vi "main screen V2.vi"() -> ()   [LabVIEW 2020]
uses:
  <vilib>/userdefined/High Color/IMAQdx.ctl
  <vilib>/DAQmx/read.llb/DAQmx Read (Analog 1D DBL NChan 1Samp).vi
  <vilib>/DAQmx/create/channels.llb/DAQmx Create Channel (AI-Voltage-Basic).vi
  <vilib>/DAQmx/create/channels.llb/DAQmx Create Channel (AI-Temperature-Thermocouple).vi
  <vilib>/DAQmx/configure/timing.llb/DAQmx Timing (Sample Clock).vi
  <vilib>/DAQmx/miscellaneous.llb/DAQmx Fill In Error Info.vi
  <vilib>/Utility/file.llb/Write Delimited Spreadsheet (string).vi
  <vilib>/Utility/file.llb/Write Delimited Spreadsheet (DBL).vi
  <vilib>/vision/driver/NI_Vision_Acquisition_Software.lvlib
  <resource>/objmgr/imaqdx.rc
  <resource>/objmgr/daqmx.rc
panel:
  out "Saving Data":bool
  out "System Time":dbl
  in  "Sample Rate":dbl=90.0
  out "error out 2":errorcluster
  out "Image 2":T1(plugin-control)
  out "Image":T1(plugin-control)
  out "error out":errorcluster
  out "Clock":dbl[](graph)
  out "T.C 2":dbl[](graph)
  out "T.C 3":dbl[](graph)
  out "T.C 4":dbl[](graph)
  out "T.C 5":dbl[](graph)
  out "T.C 6":dbl[](graph)
  out "T.C 7":dbl[](graph)
  out "Front Diode":dbl[](graph)
  out "Rear Diode":dbl[](graph)
  out "T.C 1":dbl[](graph)
  out "T.C 8":dbl[](graph)
  in  "stop":bool
  in  "physical channels":tag="cDAQ1Mod1/ai1,cDAQ1Mod1/ai2"
  in  "TC channel":tag="cDAQ1Mod3/ai0,cDAQ1Mod3/ai1,cDAQ1Mod3/ai2,cDAQ1Mod3/ai3,cDAQ1Mod3/ai4,cDAQ1Mod3/ai5,cDAQ1Mod3/ai6,cDAQ1Mod3/ai7"
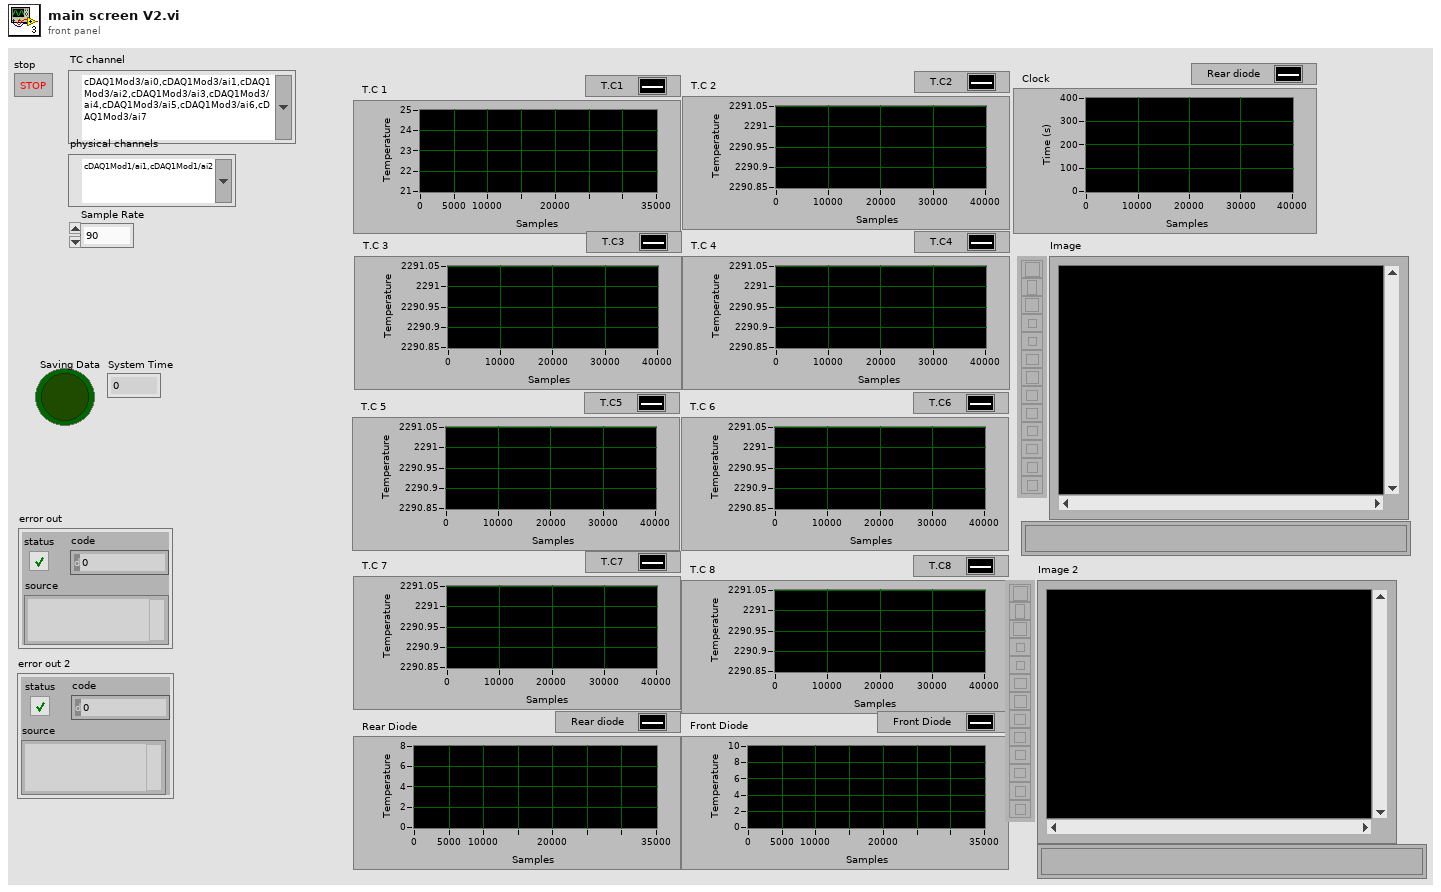
[diagram p1: front panel]
types:
  T1 = typedef "IMAQ Image.ctl" = refnum<image>
  T2 = typedef "IMAQdx.ctl" = refnum<k21>
  T3 = typedef "IMAQ AVI2 Refnum.ctl" = refnum<k20>
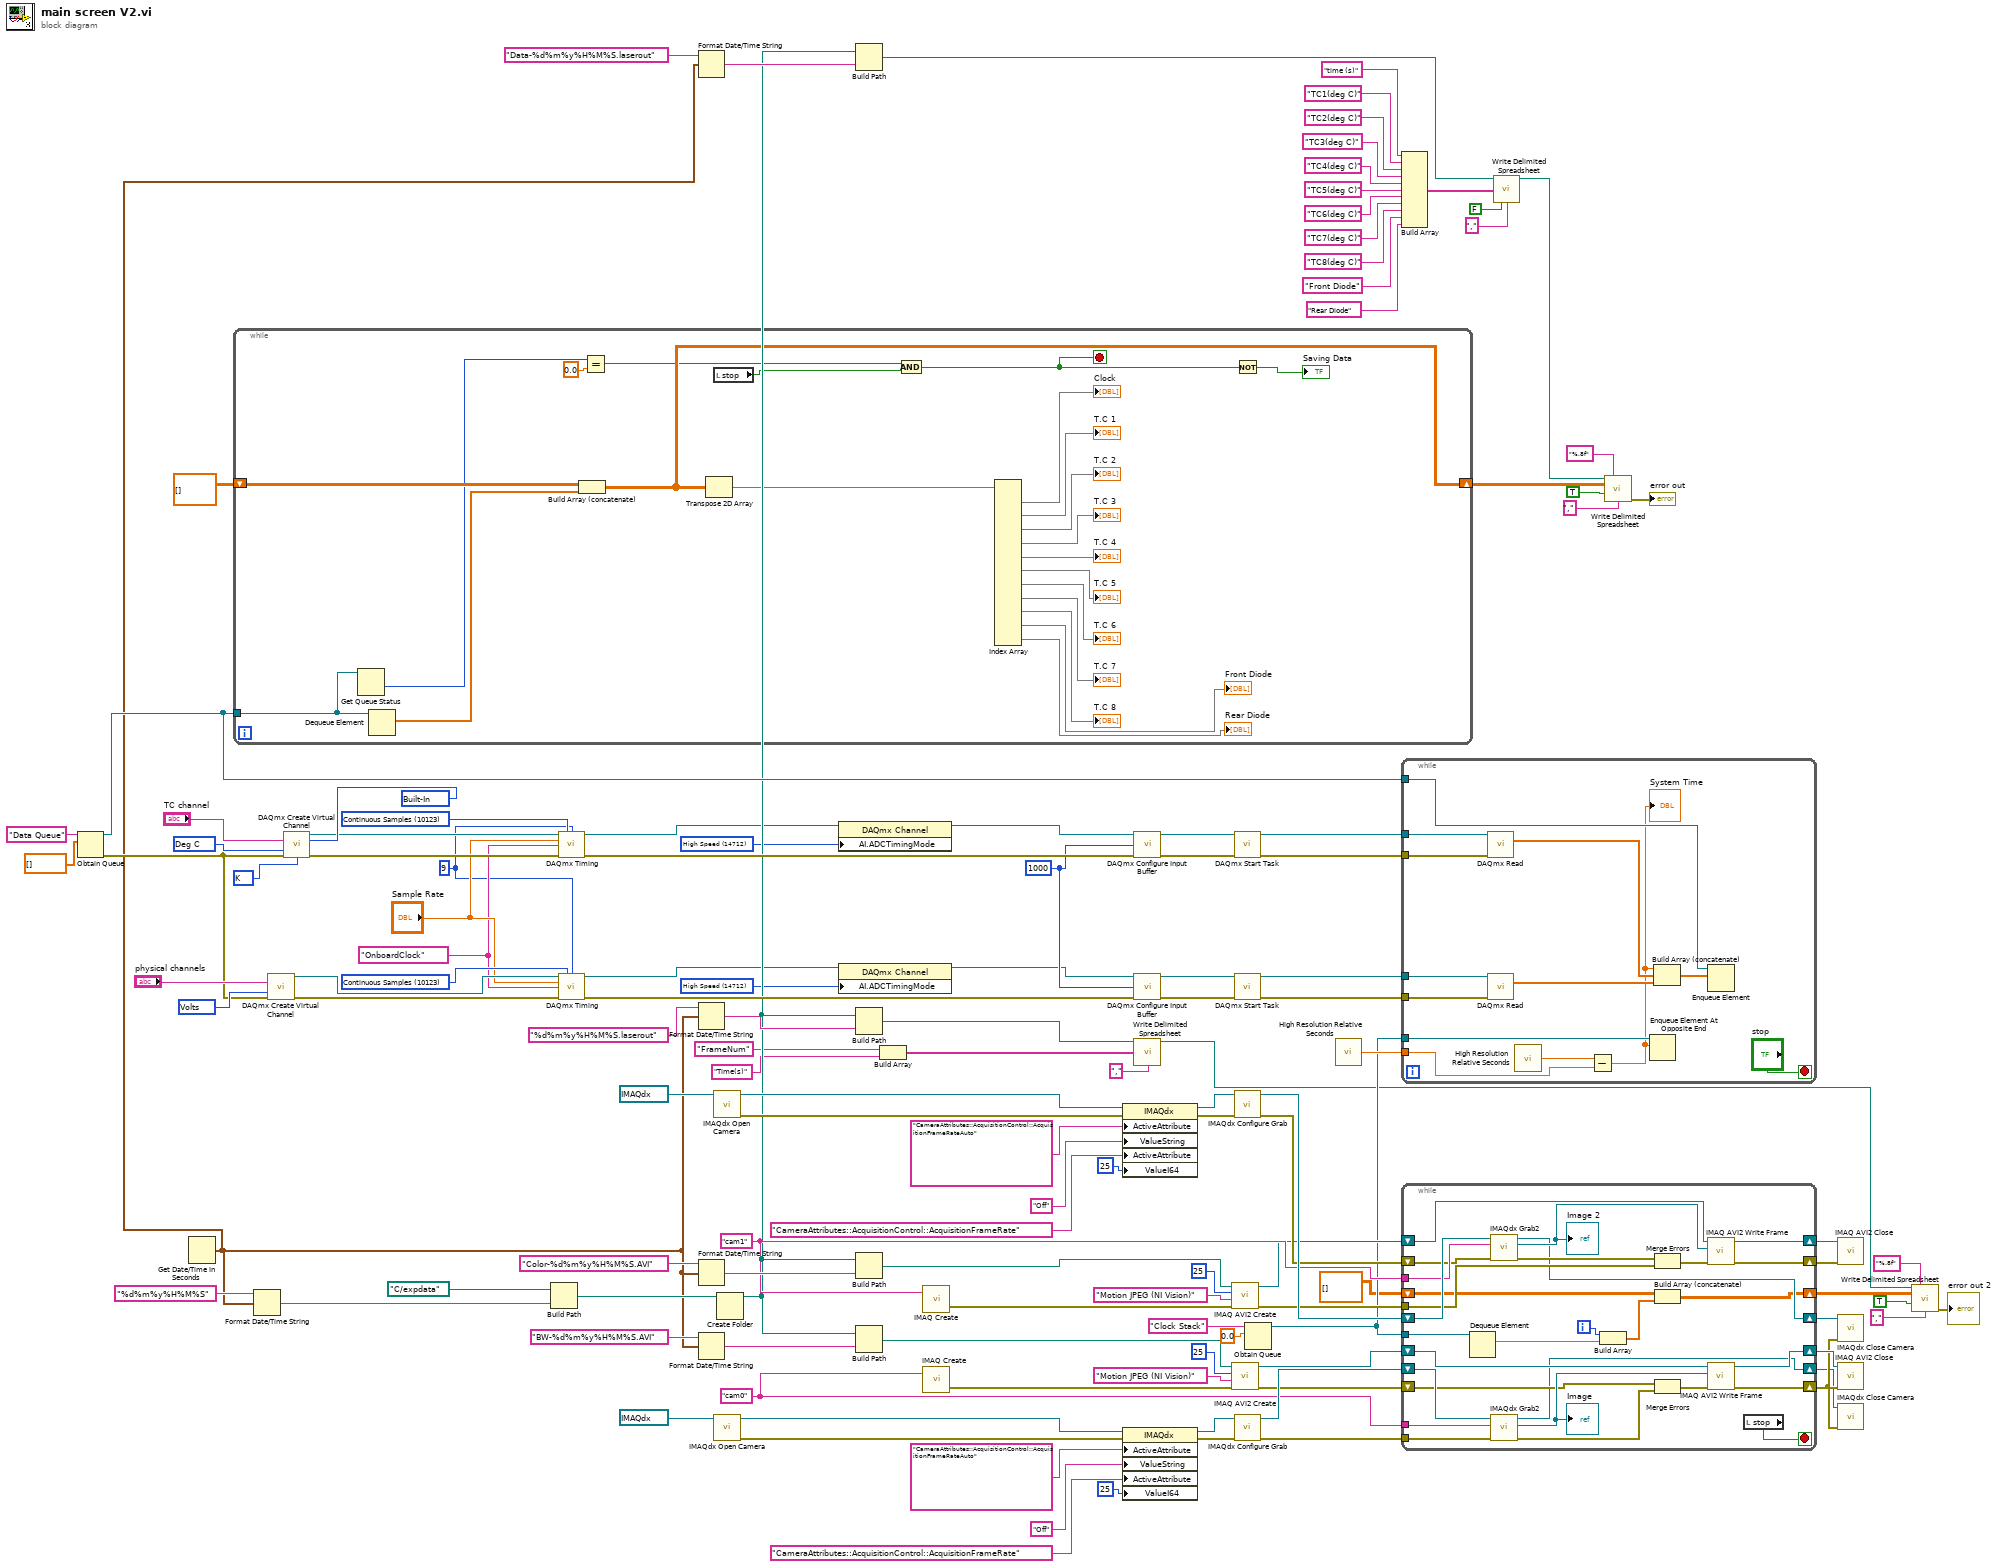
[diagram p0: block diagram]
diagram:
  w1 = 14712 items=["Automatic"=16097, "High Resolution"=10195, "High Speed"=14712, "Best 50 Hz Rejection"=14713, "Best 60 Hz Rejection"=14714, "Custom"=10137] ("AI.ADCTimingMode")
  w4 = 14712 items=["Automatic"=16097, "High Resolution"=10195, "High Speed"=14712, "Best 50 Hz Rejection"=14713, "Best 60 Hz Rejection"=14714, "Custom"=10137] ("AI.ADCTimingMode")
  w7 = 9 ("samples per channel")
  w8 = tag "OnboardClock" ("source")
  w44 = "cam1" ("Image Name")
  w38 = "cam0" ("Image Name")
  w105 = u32 1000 ("buffer size (in samples per channel)")
  w117 = 10123 items=["Finite Samples"=10178, "Continuous Samples"=10123, "Hardware Timed Single Point"=12522] ("sample mode")
  w118 = 10123 items=["Finite Samples"=10178, "Continuous Samples"=10123, "Hardware Timed Single Point"=12522] ("sample mode")
  w119 = 10073 items=["J"=10072, "K"=10073, "N"=10077, "R"=10082, "S"=10085, "T"=10086, "B"=10047, "E"=10055] ("thermocouple type")
  w123 = 10348 items=["Volts"=10348, "From Custom Scale"=10065] ("units")
  w125 = 10200 items=["Built-In"=10200, "Constant Value"=10116, "Channel"=10113] ("cjc source")
  w126 = 10143 items=["Deg C"=10143, "Deg F"=10144, "Kelvins"=10325, "Deg R"=10145, "From Custom Scale"=10065] ("units")
  n1 = Obtain Queue(name (unnamed)="Data Queue", element data type=dbl[] []) -> (queue out=w130:refnum<queue>, error out=w77:errorcluster)  [unwired: 3 in, 1 out]
  n2 = Get Date/Time In Seconds() -> (seconds since 1Jan1904=w25:timestamp)
  n3 = while {
    tunnel: w130 -> [w135]
    shift-right: [w139] -> w80
    shift-left: dbl[][] [] -> [w152]
    stop <- w132 stop-if-true
    n4 = Get Queue Status(queue=w135) -> (# pending insert=w134:i32)  [unwired: 2 in, 7 out]
    n5 = Dequeue Element(queue=w135) -> (element=w151:dbl[])  [unwired: 2 in, 3 out]
    n6 = Build Array (concatenate)(w152, w151) -> (w139:dbl[][])
    n7 = Equal?(x=w134, y=0.0) -> (x = y?=w137:bool)
    n8 = Transpose 2D Array(2D array=w139) -> (transposed array=w138:dbl[][])
    n9 = local read "stop"() -> (w133:bool)
    n10 = And(x=w137, y=w133) -> (x .and. y?=w132:bool)
    n11 = Index Array(array=w138) -> (element #1=→"Clock":dbl[], element #2=→"T.C 1":dbl[], element #3=→"T.C 2":dbl[], element #4=→"T.C 3":dbl[], element #5=→"T.C 4":dbl[], element #6=→"T.C 5":dbl[], element #7=→"T.C 6":dbl[], element #8=→"T.C 7":dbl[], element #9=→"T.C 8":dbl[], element #10=→"Front Diode":dbl[], element #11=→"Rear Diode":dbl[])  [unwired: 22 in]
    n12 = Not(x=w132) -> (.not. x?=→"Saving Data":bool)
  }
  n13 = Format Date/Time String(time format string (%c)="%d%m%y%H%M%S", seconds (now)=w25) -> (date/time string=w101:string)  [unwired: 1 in]
  n14 = call-poly <vilib>:"DAQmx Create Virtual Channel.vi"("physical channels"="physical channels", "units"=w123, "error in"=w77) -> ("task out"=w122:refnum<k21>, "error out"=w76:errorcluster)  [unwired: 11 in]
  n15 = call-poly <vilib>:"DAQmx Create Virtual Channel.vi"("physical channels"="TC channel", "cjc source"=w125, "units"=w126, "error in"=w77, "thermocouple type"=w119) -> ("task out"=w121:refnum<k21>, "error out"=w120:errorcluster)  [unwired: 9 in]
  n16 = Build Path(base path=path "C:/expdata", name or relative path=w101) -> (appended path=w100:path)
  n17 = call-poly <vilib>:"DAQmx Timing.vi"("task/channels in"=w121, "sample mode"=w118, "samples per channel"=w7, "rate"="Sample Rate", "source"=w8, "error in"=w120) -> ("task out"=w3:refnum<k21>, "error out"=w115:errorcluster)  [unwired: 8 in]
  n18 = call-poly <vilib>:"DAQmx Timing.vi"("task/channels in"=w122, "sample mode"=w117, "samples per channel"=w7, "rate"="Sample Rate", "source"=w8, "error in"=w76) -> ("task out"=w6:refnum<k21>, "error out"=w116:errorcluster)  [unwired: 8 in]
  n19 = Format Date/Time String(time format string (%c)="Data-%d%m%y%H%M%S.laserout", seconds (now)=w25) -> (date/time string=w98:string)  [unwired: 1 in]
  n20 = Format Date/Time String(time format string (%c)="%d%m%y%H%M%S.laserout", seconds (now)=w25) -> (date/time string=w24:string)  [unwired: 1 in]
  n21 = Format Date/Time String(time format string (%c)="Color-%d%m%y%H%M%S.AVI", seconds (now)=w25) -> (date/time string=w49:string)  [unwired: 1 in]
  n22 = Format Date/Time String(time format string (%c)="BW-%d%m%y%H%M%S.AVI", seconds (now)=w25) -> (date/time string=w52:string)  [unwired: 1 in]
  n23 = call <vilib>:"IMAQdx Open Camera.vi"("Session In"=T2 "cam1") -> ("error out"=w63:errorcluster, "Session Out"=w65:T2)  [unwired: 9 in]
  n24 = call <vilib>:"IMAQdx Open Camera.vi"("Session In"=T2 "cam0") -> ("error out"=w72:errorcluster, "Session Out"=w74:T2)  [unwired: 9 in]
  n25 = Create Folder(path (use dialog)=w100) -> (created path=w23:path)  [unwired: 2 in, 2 out]
  n26 = property class="DAQmx Channel"(reference=w3, "AI.ADCTimingMode"=w1) -> (reference out=w2:refnum<k21>)  [unwired: 1 in, 1 out]
  n27 = property class="DAQmx Channel"(reference=w6, "AI.ADCTimingMode"=w4) -> (reference out=w5:refnum<k21>)  [unwired: 1 in, 1 out]
  n28 = Build Path(base path=w23, name or relative path=w98) -> (appended path=w86:path)
  n29 = Build Path(base path=w23, name or relative path=w24) -> (appended path=w22:path)
  n30 = Build Path(base path=w23, name or relative path=w49) -> (appended path=w48:path)
  n31 = Build Path(base path=w23, name or relative path=w52) -> (appended path=w51:path)
  n32 = Build Array("FrameNum", "Time(s)") -> (w18:string[])
  n33 = call "IMAQ Create"("Image Name"=w44) -> ("error out"=w56:errorcluster)  [unwired: 4 in, 1 out]
  n34 = call "IMAQ Create"("Image Name"=w38) -> ("error out"=w55:errorcluster)  [unwired: 4 in, 1 out]
  n35 = property class="IMAQdx"(reference=w65, error in=w63, "ActiveAttribute"="CameraAttributes::AcquisitionControl::AcquisitionFrameRateAuto", "ValueString"="Off", "ActiveAttribute"="CameraAttributes::AcquisitionControl::AcquisitionFrameRate", "ValueI64"=u32 25 ("ValueU32")) -> (reference out=w64:T2, error out=w62:errorcluster)
  n36 = property class="IMAQdx"(reference=w74, error in=w72, "ActiveAttribute"="CameraAttributes::AcquisitionControl::AcquisitionFrameRateAuto", "ValueString"="Off", "ActiveAttribute"="CameraAttributes::AcquisitionControl::AcquisitionFrameRate", "ValueI64"=u32 25 ("ValueU32")) -> (reference out=w73:T2, error out=w71:errorcluster)
  n37 = call <vilib>:"DAQmx Configure Input Buffer.vi"("task/channels in"=w2, "buffer size (in samples per channel)"=w105, "error in"=w115) -> ("task out"=w113:refnum<k21>, "error out"=w111:errorcluster)  [unwired: 11 in]
  n38 = call <vilib>:"DAQmx Configure Input Buffer.vi"("task/channels in"=w5, "buffer size (in samples per channel)"=w105, "error in"=w116) -> ("task out"=w109:refnum<k21>, "error out"=w106:errorcluster)  [unwired: 11 in]
  n39 = call-poly <vilib>:"Write Delimited Spreadsheet.vi"("file path (dialog if empty)"=w22, "1D data"=w18, "delimiter (\\t)"="," ("delimiter (\\t)")) -> ("new file path (Not A Path if cancelled)"=w14:path)  [unwired: 11 in, 1 out]
  n40 = call "IMAQ AVI2 Create"("error in (no error)"=w56, "Codec"="Motion JPEG (NI Vision)", "Frames Per Second"=u32 25, "AVI Path"=w48) -> ("error out"=w41:errorcluster, "AVI Refnum"=w42:T3)  [unwired: 6 in]
  n41 = call "IMAQ AVI2 Create"("error in (no error)"=w55, "Codec"="Motion JPEG (NI Vision)", "Frames Per Second"=u32 25, "AVI Path"=w51) -> ("error out"=w36:errorcluster, "AVI Refnum"=w37:T3)  [unwired: 6 in]
  n42 = call <vilib>:"DAQmx Start Task.vi"("task/channels in"=w113, "error in"=w111) -> ("task out"=w112:refnum<k21>, "error out"=w110:errorcluster)  [unwired: 12 in]
  n43 = call <vilib>:"DAQmx Start Task.vi"("task/channels in"=w109, "error in"=w106) -> ("task out"=w108:refnum<k21>, "error out"=w107:errorcluster)  [unwired: 12 in]
  n44 = call <vilib>:"IMAQdx Configure Grab.vi"("error in"=w62, "Session In"=w64) -> ("error out"=w43:errorcluster, "Session Out"=w45:T2)  [unwired: 8 in]
  n45 = call <vilib>:"IMAQdx Configure Grab.vi"("error in"=w71, "Session In"=w73) -> ("error out"=w39:errorcluster, "Session Out"=w40:T2)  [unwired: 8 in]
  n46 = Obtain Queue(name (unnamed)="Clock Stack", element data type=0.0) -> (queue out=w27:refnum<queue>)  [unwired: 3 in, 2 out]
  n47 = call <vilib>:"High Resolution Relative Seconds.vi"() -> ("relative seconds"=w114:dbl)
  n48 = Build Array("time (s)", "TC1(deg C)", "TC2(deg C)", "TC3(deg C)", "TC4(deg C)", "TC5(deg C)", "TC6(deg C)", "TC7(deg C)", "TC8(deg C)", "Front Diode", "Rear Diode") -> (w85:string[])
  n49 = while {
    tunnel: w130 -> [w165]
    tunnel: w112 -> [w164]
    tunnel: w110 -> [w163]
    tunnel: w108 -> [w162]
    tunnel: w107 -> [w161]
    tunnel: w114 -> [w160]
    tunnel: w27 -> [w154]
    stop <- "stop" stop-if-true
    n50 = call-poly <vilib>:"DAQmx Read.vi"("task/channels in"=w164, "error in"=w163) -> ("data"=w158:dbl[])  [unwired: 11 in, 2 out]
    n51 = call-poly <vilib>:"DAQmx Read.vi"("task/channels in"=w162, "error in"=w161) -> ("data"=w157:dbl[])  [unwired: 11 in, 2 out]
    n52 = call <vilib>:"High Resolution Relative Seconds.vi"() -> ("relative seconds"=w159:dbl)
    n53 = Subtract(x=w159, y=w160) -> (x-y=w153:dbl)
    "System Time" <- w153
    n54 = Enqueue Element At Opposite End(queue=w154, element=w153) -> ()  [unwired: 2 in, 3 out]
    n55 = Build Array (concatenate)(w153, w158, w157) -> (w156:dbl[])
    n56 = Enqueue Element(queue=w165, element=w156) -> ()  [unwired: 2 in, 3 out]
  }
  n57 = while {
    tunnel: w44 -> [w191]
    tunnel: w41 -> [w186]
    tunnel: w39 -> [w184]
    tunnel: w38 -> [w183]
    shift-right: [w174] -> w31
    shift-left: w45 -> [w192]
    shift-right: [w176] -> w33
    shift-left: w43 -> [w190]
    shift-right: [w178] -> w35
    shift-left: w42 -> [w189]
    shift-right: [w173] -> w30
    shift-left: w40 -> [w185]
    shift-right: [w177] -> w34
    shift-left: w37 -> [w182]
    shift-right: [w175] -> w32
    shift-left: w36 -> [w180]
    tunnel: w27 -> [w172]
    shift-right: [w169] -> w13
    shift-left: dbl[][] [] -> [w170]
    i -> [w167]
    stop <- w168 stop-if-true
    n58 = Dequeue Element(queue=w172) -> (element=w166:dbl)  [unwired: 2 in, 3 out]
    n59 = call <vilib>:"IMAQdx Grab2.vi"("error in"=w190, "Image In"=w191, "Session In"=w192) -> ("error out"=w187:errorcluster, "Image Out"=w193:T1, "Session Out"=w174:T2)  [unwired: 5 in, 1 out]
    "Image 2" <- w193
    n60 = call <vilib>:"IMAQdx Grab2.vi"("error in"=w184, "Image In"=w183, "Session In"=w185) -> ("error out"=w181:errorcluster, "Image Out"=w194:T1, "Session Out"=w173:T2)  [unwired: 5 in, 1 out]
    "Image" <- w194
    n61 = Build Array(w167, w166) -> (w171:dbl[])
    n62 = Merge Errors(w187, w186) -> (w188:errorcluster)
    n63 = Build Array (concatenate)(w170, w171) -> (w169:dbl[][])
    n64 = Merge Errors(w180, w181) -> (w179:errorcluster)
    n65 = call "IMAQ AVI2 Write Frame"("error in (no error)"=w188, "Image"=w193, "AVI Refnum"=w189) -> ("error out"=w176:errorcluster, "AVI Refnum (duplicate)"=w178:T3)  [unwired: 6 in, 1 out]
    n66 = call "IMAQ AVI2 Write Frame"("error in (no error)"=w179, "Image"=w194, "AVI Refnum"=w182) -> ("error out"=w175:errorcluster, "AVI Refnum (duplicate)"=w177:T3)  [unwired: 6 in, 1 out]
    n67 = local read "stop"() -> (w168:bool)
  }
  n68 = call-poly <vilib>:"Write Delimited Spreadsheet.vi"("file path (dialog if empty)"=w86, "1D data"=w85, "transpose? (no:F)"=FALSE, "delimiter (\\t)"="," ("delimiter (\\t)")) -> ("new file path (Not A Path if cancelled)"=w79:path)  [unwired: 10 in, 1 out]
  n69 = call-poly <vilib>:"Write Delimited Spreadsheet.vi"("file path (dialog if empty)"=w79, "format (%.3f)"="%.8f", "2D data"=w80, "append to file? (new file:F)"=TRUE, "delimiter (\\t)"="," ("delimiter (\\t)")) -> ("error out"=→"error out":errorcluster)  [unwired: 9 in, 1 out]
  n70 = call "IMAQ AVI2 Close"("error in (no error)"=w33, "AVI Refnum"=w35) -> ()  [unwired: 9 in, 1 out]
  n71 = call <vilib>:"IMAQdx Close Camera.vi"("error in"=w32, "Session In"=w31) -> ()  [unwired: 9 in, 1 out]
  n72 = call "IMAQ AVI2 Close"("error in (no error)"=w32, "AVI Refnum"=w34) -> ()  [unwired: 9 in, 1 out]
  n73 = call <vilib>:"IMAQdx Close Camera.vi"("error in"=w32, "Session In"=w30) -> ()  [unwired: 9 in, 1 out]
  n74 = call-poly <vilib>:"Write Delimited Spreadsheet.vi"("file path (dialog if empty)"=w14, "format (%.3f)"="%.8f", "2D data"=w13, "append to file? (new file:F)"=TRUE, "delimiter (\\t)"="," ("delimiter (\\t)")) -> ("error out"=→"error out 2":errorcluster)  [unwired: 9 in, 1 out]
